vi "Test No Match.vi"(8 "error in (no error)":errorcluster, 11 "Test Case In":refnum<class "Pattern Matching Comparator Test.lvclass">) -> (0 "error out":errorcluster, 3 "Test Case Out":refnum<class "Pattern Matching Comparator Test.lvclass">)   [LabVIEW 2020, in "Pattern Matching Comparator Test.lvclass"]
uses:
  Pattern Matching Comparator Test.lvclass
  C:/Program Files (x86)/National Instruments/LabVIEW 2020/vi.lib/Astemes/LUnit/Test Case.lvclass
  <vilib>/Astemes/LUnit/Test Case.lvclass/Test Case.ctl
  <vilib>/Astemes/LUnit/Append Pass Result.vi
  <vilib>/Astemes/LUnit/Append Fail Result.vi
  Test Doubles/Mock VI Call/Mock VI Call.lvclass
  C:/git/astemes-lmock/source/Core/VI Call/VI Call.lvclass
  source/Comparators/String Argument Matching Comparator/String Input Matching Comparator.lvclass
  <vilib>/Astemes/LUnit/Test Case.lvclass
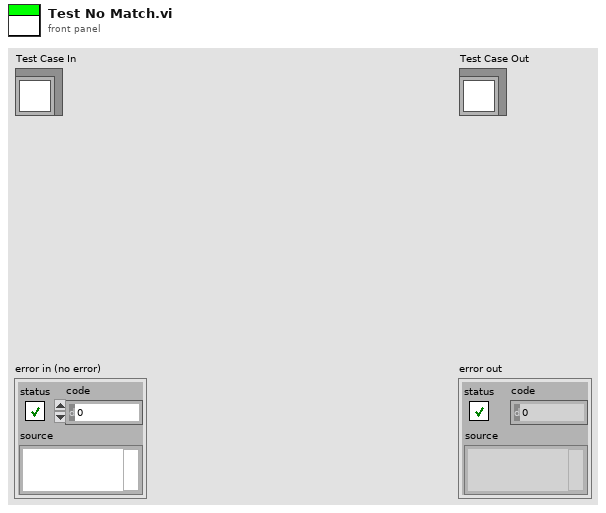
[diagram p1: front panel]
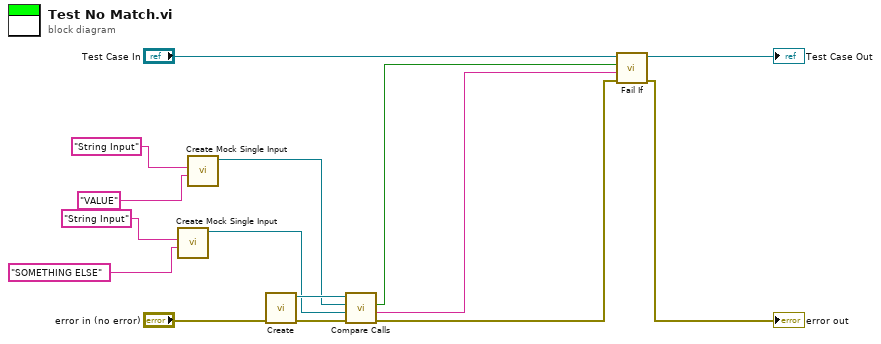
[diagram p0: block diagram]
diagram:
  n1 = call "Create Mock Single Input.vi"("Control value"="SOMETHING ELSE" ("Control Label"), "Control Label"="String Input") -> ("Mock VI Call Out"=w1:refnum<class "Mock VI Call.lvclass">)  [unwired: 8 in, 1 out]
  n2 = call "Create Mock Single Input.vi"("Control value"="VALUE" ("Control Label"), "Control Label"="String Input") -> ("Mock VI Call Out"=w8:refnum<class "Mock VI Call.lvclass">)  [unwired: 8 in, 1 out]
  n3 = call "Create.vi"("error in (no error)"="error in (no error)") -> ("error out"=w11:errorcluster, "String Argument Matching Comparator"=w12:refnum<class "String Input Matching Comparator.lvclass">)  [unwired: 9 in]
  n4 = call-dynamic "Compare Calls.vi"("error in (no error)"=w11, "VI Call 2"=w1, "VI Call 1"=w8, "String Argument Matching Comparator in"=w12) -> ("error out"=w4:errorcluster, "Description"=w6:string, "Equal?"=w7:bool)  [unwired: 5 in]
  n5 = call <vilib>:"Fail If.vi"("error in (no error)"=w4, "Message"=w6, "Fail?"=w7, "LUnit Test Case In"="Test Case In") -> ("error out"=→"error out":errorcluster, "LUnit Test Case Out"=→"Test Case Out":refnum<class "Pattern Matching Comparator Test.lvclass">)  [unwired: 6 in]
